vi "Add VIs to Library.vi"(8 "error in":errorcluster, 11 "Library":refnum<vi>) -> (0 "error out":errorcluster, 3 "Library out":refnum<vi>)   [LabVIEW 2020, in "WebServiceImporter.lvlib" / "VI Generator.lvlib"]
uses:
  <vilib>/Platform/WebService/VI Generator/VI Generator.lvlib
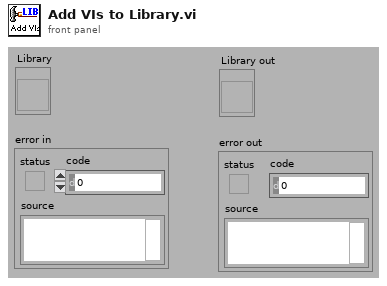
[diagram p1: front panel]
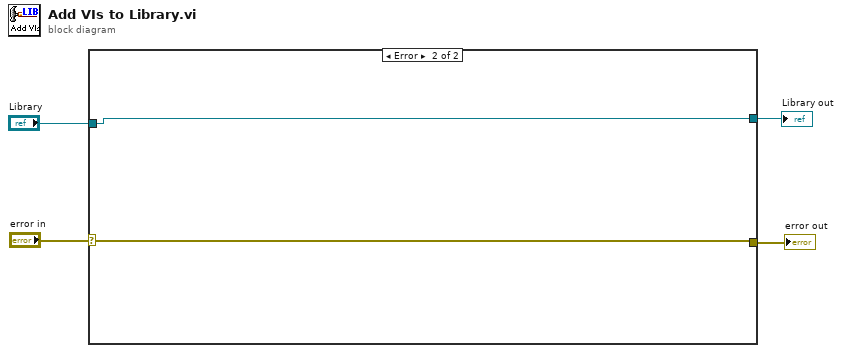
[diagram p0: block diagram]
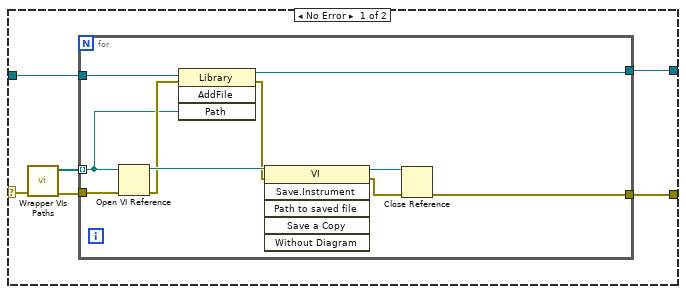
[diagram p2: hidden frame]
diagram:
  n1 = case shown="Error" "error in" {
    selector: "error in" -> [w8 w21]
    tunnel: "Library" -> [w9 w22]
    tunnel: [w6 w21] -> w2
    tunnel: [w5 w22] -> w1
    frame No Error {
      n2 = call <vilib>:"Wrapper VIs Paths.vi"("error in (no error)"=w8) -> ("error out"=w7:errorcluster, "Array"=w10:path[])  [unwired: 9 in]
      n3 = for {
        tunnel: w10 -> [w17] mode=indexing
        tunnel: w9 -> [w16]
        tunnel: w7 -> [w20]
        tunnel: [w12] -> w6
        tunnel: [w11] -> w5
        n4 = Open VI Reference(vi path=w17, error in (no error)=w20) -> (vi reference=w19:refnum<vi>, error out=w18:errorcluster)  [unwired: 4 in]
        n5 = invoke class="Library" method="AddFile"(reference=w16, error in=w18, "Path"=w17) -> (reference out=w11:refnum<vi>, error out=w15:errorcluster)  [unwired: 1 in, 2 out]
        n6 = invoke class="VI" method="Save.Instrument"(reference=w19, error in=w15) -> (reference out=w14:refnum<vi>, error out=w13:errorcluster)  [unwired: 4 in, 4 out]
        n7 = Close Reference(reference=w14, error in (no error)=w13) -> (error out=w12:errorcluster)
      }
    }
    frame Error {
    }
  }
  "error out" <- w2
  "Library out" <- w1
